vi "UHR-Fleezers Control (host) -Leonardo 04-2018 V1.vi"(0 "Tab Control":T5(tab)=enum."Trap Control (RF)") -> ()   [LabVIEW 2013] (continued)
        n483 = property on="APD Chart" class="WFChart (strict)"("YScale.Maximum"=w830) -> ()  [unwired: 2 in, 2 out]
      }
      event "Phase adj. (AI1)", "+ phase (AI1)", "- phase (AI1)": Value Change {
        n484 = event-data() -> ()  [unwired: 7 out]
        n485 = Negate(x="Phase adj. (AI1)") -> (-x=w847:i16)
        n486 = Select(t=w847, s="- phase (AI1)", f="Phase adj. (AI1)") -> (s? t:f=w846:i16)
        n487 = xnode "Read/Write Control"("FPGA VI Reference In"=w850, "error in"=w849, "Phase count adjustment"=w846) -> ("FPGA VI Reference Out"=w845:T20, "error out"=w844:errorcluster)
        n488 = Or(x="- phase (AI1)", y="+ phase (AI1)") -> (x .or. y?=w841:bool)
        n489 = xnode "Read/Write Control"("FPGA VI Reference In"=w845, "error in"=w844, "+ phase"=w841) -> ("error out"=w840:errorcluster)  [unwired: 1 out]
      }
      event "Signals to Plot": Double Click {
        w853 = u32 9868950 ("Color Box")
        n490 = event-data() -> ("Row"=w855:i32)  [unwired: 9 out]
        n491 = property on="All Signals" class="WFChart (strict)"("Active Plot"=w855) -> (error out=w866:errorcluster)  [unwired: 2 in, 1 out]
        n492 = property on="All Signals" class="WFChart (strict)" props=["Plot", "Visible?", "Plot", "Plot Color"](error in=w866) -> (error out=w865:errorcluster, "Plot.Visible?"=w864:bool)  [unwired: 1 in, 2 out]
        n493 = Select(t=FALSE ("Plot.Visible"), s=w864, f=TRUE ("Plot.Visible")) -> (s? t:f=w859:bool)
        n494 = property on="All Signals" class="WFChart (strict)"(error in=w865, "Plot.Visible?"=w859) -> (error out=w861:errorcluster)  [unwired: 1 in, 1 out]
        n495 = property on="All Signals" class="WFChart (strict)"(error in=w861) -> (error out=w856:errorcluster, "Plot.Plot Color"=w860:u32)  [unwired: 1 in, 1 out]
        n496 = property on="Signals to Plot" class="LstBox (strict)"(error in=w856, "Active Row"=w855) -> (error out=w854:errorcluster)  [unwired: 1 in, 1 out]
        n497 = Select(t=w860, s=w859, f=u32 0) -> (s? t:f=w857:u32)
        n498 = property on="Signals to Plot" class="LstBox (strict)"(error in=w854, "CellFontColor"=w857, "SelColor"=w853, "CellBG"=w853, "CellFontSize"=u32 20 ("Active Row:Cell Font:Size"), "CellFontBold"=TRUE ("Active Row:Cell Font:Bold")) -> ()  [unwired: 1 in, 2 out]
      }
      event "Dynamic Force FB": Value Change {
        n499 = event-data() -> ()  [unwired: 7 out]
        n500 = xnode "Read/Write Control"("FPGA VI Reference In"=w868, "Dynamic Force FB (Ronen)"="Dynamic Force FB") -> ()  [unwired: 1 in, 2 out]
      }
      event "BD 1 Frequency 1 (MHz)", "BD 1 Frequency 2 (MHz)", "BD 1 Frequency 3 (MHz)", "BD 2 Frequency 1 (MHz)", "BD 2 Frequency 2 (MHz)", "BD 2 Frequency 3 (MHz)", "Trap Delta (MHz)": Value Change {
        # "anytime one of the frequencies is changed, write it to the RF board UNLESS Set 2 is being oscillated. The oscillation\nscript writes the frequencies to the RF board."
        n501 = event-data() -> ("CtlRef"=w871:refnum<vi>)  [unwired: 6 out]
        n502 = control-ref of="Trap Delta (MHz)"() -> (w870:refnum<vi>)
        n503 = Equal?(x=w870, y=w871) -> (x = y?=w869:bool)
        n504 = case shown="False" "Oscillate Set 2" {
          tunnel: w874 -> [w895 _]
          tunnel: [w894 w907] -> w873
          tunnel: w872 -> [w893 w907]
          tunnel: w869 -> [w880 _]
          frame False {
            n505 = case shown="True" "Symmetric manual \ntrap motion" {
              tunnel: ["T2 for asymmetric\n(MHz)" w906] -> w881
              tunnel: "Trap Delta (MHz)" -> [w900 w905]
              tunnel: [w899 w902] -> w877
              frame False {
                n506 = Subtract(x="T2 for asymmetric\n(MHz)", y=w900) -> (x-y=w899:dbl)
              }
              frame True {
                n507 = Divide(x=w905, y=2) -> (x/y=w903:dbl)
                n508 = Subtract(x="Middle freq for \nsymmetric (MHz)", y=w903) -> (x-y=w902:dbl)
                n509 = Add(x="Middle freq for \nsymmetric (MHz)", y=w903) -> (x+y=w906:dbl)
              }
            }
            n510 = local read "BD 1 Frequency 2 (MHz)"() -> (w882:dbl)
            n511 = local write "BD 1 Frequency 1 (MHz)"(w877) -> ()
            n512 = Select(t=w881, s=w880, f=w882) -> (s? t:f=w879:dbl)
            n513 = local read "Y RF Frequency Limits (MHz)"() -> (w883:T16)
            n514 = local read "X RF Frequency Limits (MHz)"() -> (w884:T16)
            n515 = local read "BD 1 Frequency 3 (MHz)"() -> (w896:dbl)
            n516 = local write "BD 1 Frequency 2 (MHz)"(w879) -> ()
            n517 = local read "BD 2 Frequency 1 (MHz)"() -> (w887:dbl)
            n518 = local read "BD 2 Frequency 2 (MHz)"() -> (w886:dbl)
            n519 = local read "BD 2 Frequency 3 (MHz)"() -> (w897:dbl)
            n520 = call "set RF board frequency - interlace.vi"("Board 2 Frequency Limits"=w883, "Board 1 Frequency Limits"=w884, "error in"=w893, "FPGA VI Reference In"=w895, "Board 2 Frequency 3 (MHz)"=w897, "Board 1 Frequency 3 (MHz)"=w896, "Board 2 Frequency 2 (MHz)"=w886, "Board 2 Frequency 1 (MHz)"=w887, "Board 1 Frequency 2 (MHz)"=w879, "Board 1 Frequency 1  (MHz)"=w877) -> ("error out"=w894:errorcluster)  [unwired: 1 out]
            n521 = Subtract(x=w887, y=w886) -> (x-y=w891:dbl)
            n522 = Subtract(x=w879, y=w877) -> (x-y=w892:dbl)
            n523 = Square(x=w891) -> (x^2=w889:dbl)
            n524 = Square(x=w892) -> (x^2=w890:dbl)
            n525 = Add(x=w890, y=w889) -> (x+y=w888:dbl)
            n526 = Square Root(x=w888) -> (sqrt(x)=w885:dbl)
            n527 = local write "Trap Delta (MHz)"(w885) -> ()
            n528 = property on="Initial delta (MHz)" class="DigNum (strict)"("Val(Sgnl)"=w885) -> ()  [unwired: 2 in, 2 out]
          }
          frame True {
          }
        }
      }
      event "Round T1 X": Value Change {
        n529 = event-data() -> ()  [unwired: 7 out]
        n530 = local read "BD 1 Frequency 1 (MHz)"() -> (w910:dbl)
        n531 = Round To Nearest(number=w910) -> (nearest integer value=w909:dbl)
        n532 = property on="BD 1 Frequency 1 (MHz)" class="DigNum (strict)"("Val(Sgnl)"=w909) -> ()  [unwired: 2 in, 2 out]
      }
      event "Round T2 X": Value Change {
        n533 = event-data() -> ()  [unwired: 7 out]
        n534 = local read "BD 1 Frequency 2 (MHz)"() -> (w912:dbl)
        n535 = Round To Nearest(number=w912) -> (nearest integer value=w911:dbl)
        n536 = property on="BD 1 Frequency 2 (MHz)" class="DigNum (strict)"("Val(Sgnl)"=w911) -> ()  [unwired: 2 in, 2 out]
      }
      event "Stop All": Value Change {
        n537 = event-data() -> ()  [unwired: 7 out]
        n538 = call "hamilton_controller.vi"("action"=T21."DISCONNECT") -> ()  [unwired: 10 in, 1 out]
        n539 = local read "Stop All"() -> (w915:bool)
      }
      event "Delayed Interlace Start": Value Change {
        n540 = event-data() -> ()  [unwired: 7 out]
        n541 = flat-sequence {
          frame #0 {
            n542 = Multiply(x="Delay to Interlace (s)", y=1000.0) -> (x*y=w918:dbl)
            n543 = Wait (ms)(milliseconds to wait=w918) -> ()  [unwired: 1 out]
          }
          frame #1 {
            n544 = property on="Green laser mode" class="RadioBtnsControl (strict)"("Val(Sgnl)"=enum32{"Laser ON", "Laser OFF", "Interlace"}."Interlace" ("Value (Signaling)")) -> ()  [unwired: 2 in, 2 out]
          }
        }
      }
      event "BD 1 Amplitude 1 (%)", "BD 1 Amplitude 2 (%)", "BD 1 Amplitude 3 (%)", "BD 2 Amplitude 1 (%)", "BD 2 Amplitude 2 (%)", "BD 2 Amplitude 3 (%)", "Trap 1 ON", "Trap 2 ON", "Trap 3 ON", "Feedback On/Off", "All FB On/Off": Value Change {
        w942 = i16 1 ("f")
        n545 = event-data() -> ()  [unwired: 7 out]
        n546 = local write "Trap 1 (ON/OFF)"("Trap 1 ON") -> ()
        n547 = local write "Trap 2 (ON/OFF)"("Trap 2 ON") -> ()
        n548 = Boolean To (0,1)(Boolean="Trap 3 ON") -> (0, 1=w943:i16)
        n549 = Boolean To (0,1)(Boolean="Trap 1 ON") -> (0, 1=w944:i16)
        n550 = Boolean To (0,1)(Boolean="Trap 2 ON") -> (0, 1=w945:i16)
        n551 = Select(t=w945, s="Trap ON/OFF X or Y Amp?", f=w942) -> (s? t:f=w940:i16)
        n552 = Select(t=w944, s="Trap ON/OFF X or Y Amp?", f=w942) -> (s? t:f=w941:i16)
        n553 = Select(t=w943, s="Trap ON/OFF X or Y Amp?", f=w942) -> (s? t:f=w939:i16)
        n554 = Select(t=w942, s="Trap ON/OFF X or Y Amp?", f=w945) -> (s? t:f=w937:i16)
        n555 = Select(t=w942, s="Trap ON/OFF X or Y Amp?", f=w944) -> (s? t:f=w938:i16)
        n556 = Select(t=w942, s="Trap ON/OFF X or Y Amp?", f=w943) -> (s? t:f=w936:i16)
        n557 = And(x="All FB On/Off", y="Feedback On/Off") -> (x .and. y?=w934:cluster{"Set 1":bool, "Set 2":bool})
        n558 = local read "BD 1 Amplitude 1 (%)"() -> (w954:dbl)
        n559 = local read "BD 1 Amplitude 2 (%)"() -> (w953:dbl)
        n560 = local read "BD 1 Amplitude 3 (%)"() -> (w952:dbl)
        n561 = Unbundle By Name(w934) -> ("Set 1"=w930:bool, "Set 2"=w927:bool)
        n562 = local read "Y RF Amplitude Limits (%)"() -> (w923:T16)
        n563 = local read "X RF Amplitude Limits (%)"() -> (w924:T16)
        n564 = local read "BD 2 Amplitude 1 (%)"() -> (w955:dbl)
        n565 = local read "BD 2 Amplitude 2 (%)"() -> (w956:dbl)
        n566 = local read "BD 2 Amplitude 3 (%)"() -> (w957:dbl)
        n567 = And(x="Trap 2 ON", y=w927) -> (x .and. y?=w925:bool)
        n568 = And(x="Trap 1 ON", y=w930) -> (x .and. y?=w928:bool)
        n569 = Multiply(x=w941, y=w954) -> (x*y=w949:dbl)
        n570 = Multiply(x=w953, y=w940) -> (x*y=w947:dbl)
        n571 = Multiply(x=w952, y=w939) -> (x*y=w948:dbl)
        n572 = Multiply(x=w955, y=w938) -> (x*y=w958:dbl)
        n573 = Multiply(x=w956, y=w937) -> (x*y=w959:dbl)
        n574 = Multiply(x=w957, y=w936) -> (x*y=w960:dbl)
        n575 = call "set RF board amplitude - interlace.vi"("Board 2 Amplitude Limits"=w923, "Board 1 Amplitude Limits"=w924, "error in"=w950, "FPGA VI Reference In"=w951, "Board 2 Amplitude 3 (%)"=w960, "Board 1 Amplitude 3 (%)"=w948, "Board 2 Amplitude 2 (%)"=w959, "Board 2 Amplitude 1 (%)"=w958, "Board 1 Amplitude 2 (%)"=w947, "Board 1 Amplitude 1 (%)"=w949) -> ("error out"=w932:errorcluster, "FPGA VI Reference Out"=w933:T20)
        n576 = xnode "Read/Write Control"("FPGA VI Reference In"=w933, "error in"=w932, "FB On/Off Set 1"=w928, "FB On/Off Set 2"=w925) -> ("error out"=w931:errorcluster)  [unwired: 1 out]
        n577 = case shown="True" "All FB On/Off" {
          frame False {
          }
          frame True {
            n578 = local write "Feedback overload"(FALSE) -> ()
          }
        }
      }
      event "Load parameters": Value Change {
        n579 = event-data() -> ()  [unwired: 7 out]
        n580 = property on="Saved AOD Raster Scan Parameter Sets" class="Arr (strict)"() -> ("Index Values"=w972:u32[])  [unwired: 2 in, 2 out]
        n581 = Index Array(array=w972, index=0) -> (element=w969:u32)
        n582 = local write "Load parameters"(FALSE ("Load parameters")) -> ()
        n583 = Index Array(array="Saved AOD Raster Scan Parameter Sets", index=w969) -> (element=w968:T31)
        n584 = Unbundle By Name(w968) -> ("Scan Range AOD (nm) 2"=w967:dbl, "Step Size AOD (nm) 2"=w966:dbl, "Scan Speed AOD (nm/s) 2"=w965:dbl, "Number of scans (AOD) 2"=w964:u16)
        n585 = flat-sequence {
          tunnel: w967 -> [w975]
          tunnel: w966 -> [w974]
          tunnel: w965 -> [w973]
          tunnel: w964 -> [w976]
          frame #0 {
            n586 = local write "Scan Speed (nm/s)"(w973) -> ()
            n587 = local write "Scan Range (nm)"(w975) -> ()
            n588 = local write "Step Size (nm)"(w974) -> ()
          }
          frame #1 {
            n589 = property on="Number of F/B Scans (AOD)" class="DigNum (strict)"("Val(Sgnl)"=w976) -> ()  [unwired: 2 in, 2 out]
          }
        }
      }
      event "Trap 1 (ON/OFF)", "Trap 2 (ON/OFF)": Value Change {
        n590 = event-data() -> ()  [unwired: 7 out]
        n591 = property on="Trap 2 ON" class="Bool (strict)"("Val(Sgnl)"="Trap 2 (ON/OFF)") -> ()  [unwired: 2 in, 2 out]
        n592 = property on="Trap 1 ON" class="Bool (strict)"("Val(Sgnl)"="Trap 1 (ON/OFF)") -> ()  [unwired: 2 in, 2 out]
      }
      event "DIO count 1 (ticks)", "DIO count 2 (ticks)", "DIO count 3 (ticks)", "Interlace", "Number Interlace Sets", "Not-Interlacing Set": Value Change {
        n593 = event-data() -> ()  [unwired: 7 out]
        n594 = local read "DIO count 3 (ticks)"() -> (w989:u32)
        n595 = local read "DIO count 1 (ticks)"() -> (w991:u32)
        n596 = local read "DIO count 2 (ticks)"() -> (w990:u32)
        n597 = To Unsigned Byte Integer(number="Not-Interlacing Set") -> (unsigned 8bit integer=w980:u8)
        n598 = Add(x=w980, y=u8 1) -> (x+y=w984:u8)
        n599 = xnode "Read/Write Control"("FPGA VI Reference In"=w995, "error in"=w993, "DIO count 1 (ticks)"=w991, "DIO count 2 (ticks)"=w990, "DIO count 3 (ticks)"=w989, "Interlace ON/OFF"="Interlace", "Number Interlace Cycles"="Number Interlace Sets", "Interlace Off Parameters"=w984) -> ("error out"=w994:errorcluster)  [unwired: 1 out]
        n600 = Build Array(w991, w990, w989) -> (w982:u32[])
        n601 = Split 1D Array(array=w982, index="Number Interlace Sets") -> (first subarray=w992:u32[])  [unwired: 1 out]
        n602 = Index Array(array=w982, index=w980) -> (element=w981:u32)
        n603 = Add Array Elements(numeric array=w992) -> (sum=w986:u32)
        n604 = Select(t=w986, s="Interlace", f=w981) -> (s? t:f=→"Total Counts (ticks)":u32)
      }
      event "Reset Feedback": Value Change {
        n605 = event-data() -> ()  [unwired: 7 out]
        n606 = Unbundle By Name("Reset Feedback") -> ("Set 1"=w999:bool, "Set 2"=w998:bool)
        n607 = xnode "Read/Write Control"("FPGA VI Reference In"=w1001, "error in"=w996, "FB Reset Set 1"=w999, "FB Reset Set 2"=w998) -> ("error out"=w997:errorcluster)  [unwired: 1 out]
      }
      event "PID gains": Value Change {
        n608 = event-data() -> ()  [unwired: 7 out]
        n609 = local read "PID gains"() -> (w1002:T10)
        n610 = xnode "Read/Write Control"("FPGA VI Reference In"=w1005, "error in"=w1003, "FB Gains"=w1002) -> ("error out"=w1004:errorcluster)  [unwired: 1 out]
      }
      event "AI2 to Setpoint", "Trap Intensity\nSetpoints (V)": Value Change {
        n611 = event-data() -> ()  [unwired: 7 out]
        n612 = xnode "Read/Write Control"("FPGA VI Reference In"=w1010, "error in"=w1006) -> ("FPGA VI Reference Out"=w1009:T20, "error out"=w1008:errorcluster, "AI2 Y Sum Set 1"=w1017:i16, "AI2 Y Sum Set 2"=w1016:i16)
        n613 = Cluster To Array(cluster="AI2 to Setpoint") -> (array=w1020:bool[])
        n614 = local read "AI2 (V)"() -> (w1018:cluster{"Set 1":dbl, "Set 2":dbl})
        n615 = Or Array Elements(Boolean array=w1020) -> (logical OR=w1021:bool)
        n616 = Bundle By Name(cluster=w1018, "Set 1"=w1017, "Set 2"=w1016) -> (w1015:cluster{"Set 1":dbl, "Set 2":dbl})
        n617 = Divide(x=w1015, y=3276.7) -> (x/y=w1014:cluster{"Set 1":dbl, "Set 2":dbl})
        "AI2 (V)" <- w1014
        n618 = case shown="True" w1021 {
          tunnel: [w1024 w1041] -> w1013
          tunnel: "AI2 to Setpoint" -> [_ w1037]
          tunnel: "Trap Intensity\nSetpoints (V)" -> [w1025 w1040]
          tunnel: w1014 -> [_ w1034]
          frame False {
            n619 = Multiply(x=3276.7, y=w1025) -> (x*y=w1026:cluster{"Set 1":dbl, "Set 2":dbl})
            n620 = To Word Integer(number=w1026) -> (16bit integer=w1024:cluster{"Set 1":i16, "Set 2":i16})
          }
          frame True {
            n621 = Unbundle By Name(w1034) -> ("Set 1"=w1033:dbl, "Set 2"=w1032:dbl)
            n622 = Unbundle By Name(w1040) -> ("Set 1"=w1039:dbl, "Set 2"=w1038:dbl)
            n623 = Unbundle By Name(w1037) -> ("Set 1"=w1036:bool, "Set 2"=w1035:bool)
            n624 = Select(t=w1033, s=w1036, f=w1039) -> (s? t:f=w1031:dbl)
            n625 = Select(t=w1032, s=w1035, f=w1038) -> (s? t:f=w1030:dbl)
            n626 = Bundle By Name(cluster=w1040, "Set 1"=w1031, "Set 2"=w1030) -> (w1028:cluster{"Set 1":dbl, "Set 2":dbl})
            n627 = local write "Trap Intensity\nSetpoints (V)"(w1028) -> ()
            n628 = Multiply(x=3276.7, y=w1028) -> (x*y=w1029:cluster{"Set 1":dbl, "Set 2":dbl})
            n629 = To Word Integer(number=w1029) -> (16bit integer=w1041:cluster{"Set 1":i16, "Set 2":i16})
          }
        }
        n630 = Unbundle By Name(w1013) -> ("Set 1"=w1012:i16, "Set 2"=w1011:i16)
        n631 = xnode "Read/Write Control"("FPGA VI Reference In"=w1009, "error in"=w1008, "FB Setpoint Set 1"=w1012, "FB Setpoint Set 2"=w1011) -> ("error out"=w1007:errorcluster)  [unwired: 1 out]
      }
      event "Invert GI": Value Change {
        n632 = event-data() -> ()  [unwired: 7 out]
        n633 = xnode "Read/Write Control"("FPGA VI Reference In"=w1046, "error in"=w1044, "Invert GI"="Invert GI", "Invert GI 2"="Invert GI") -> ("error out"=w1045:errorcluster)  [unwired: 1 out]
      }
      event "Green FB Setpoint (mV)", "Green FB Gains", "Green FB On/Off", "Current When FB OFF (%)", "Green int current ON count adj": Value Change {
        n634 = event-data() -> ()  [unwired: 7 out]
        n635 = local read "Green FB Setpoint (mV)"() -> (w1053:dbl)
        n636 = local read "Current When FB OFF (%)"() -> (w1056:dbl)
        n637 = Multiply(x=w1053, y=3.2767) -> (x*y=w1052:dbl)
        n638 = Multiply(x=w1056, y=655.35) -> (x*y=w1057:dbl)
        n639 = To Unsigned Word Integer(number=w1057) -> (unsigned 16bit integer=w1055:u16)
        n640 = local read "Green int current ON count adj"() -> (w1060:u32)
        n641 = local read "Green FB Gains"() -> (w1059:T10)
        n642 = local read "Green Laser ON/Interlacing"() -> (w1050:bool)
        n643 = local read "Green laser mode"() -> (w1049:enum32{"Laser ON", "Laser OFF", "Interlace"})
        n644 = local read "Green FB On/Off"() -> (w1061:bool)
        n645 = Equal?(x=w1049, y=enum32{"Laser ON", "Laser OFF", "Interlace"}."Interlace") -> (x = y?=w1047:bool)
        n646 = Compound Arithmetic op=AND(w1047, w1061, w1050) -> (w1051:bool)
        n647 = xnode "Read/Write Control"("FPGA VI Reference In"=w1064, "error in"=w1063, "Green FB Setpoint"=w1052, "Green FB On/Off"=w1051, "Current Out"=w1055, "Green int current ON count adj"=w1060, "Green FB Gains"=w1059) -> ("error out"=w1062:errorcluster)  [unwired: 1 out]
      }
      event "Green laser mode", "Green Laser ON/Interlacing": Value Change {
        n648 = event-data() -> ()  [unwired: 7 out]
        n649 = case shown="True" "Green Laser ON/Interlacing" {
          tunnel: "Green laser mode" -> [_ w1078]
          tunnel: [enum32{"Laser ON", "Laser OFF", "Interlace"}."Laser OFF" ("Green laser mode") w1078] -> w1066
          tunnel: [FALSE w1074] -> w1065
          frame False {
          }
          frame True {
            n650 = local read "Green FB On/Off"() -> (w1075:bool)
            n651 = Equal?(x=w1078, y=enum32{"Laser ON", "Laser OFF", "Interlace"}."Interlace") -> (x = y?=w1076:bool)
            n652 = And(x=w1076, y=w1075) -> (x .and. y?=w1074:bool)
          }
        }
        n653 = xnode "Read/Write Control"("FPGA VI Reference In"=w1071, "error in"=w1069, "Operating Mode"=w1066, "Operating Mode 2"=w1066, "Green FB On/Off"=w1065) -> ("error out"=w1070:errorcluster)  [unwired: 1 out]
      }
      event "- phase (APD 1 Gate)", "+ phase (APD 1 Gate)": Value Change {
        n654 = event-data() -> ()  [unwired: 7 out]
        n655 = local read "Phase Adj. (APD 1 Gate)"() -> (w1079:i16)
        n656 = Negate(x=w1079) -> (-x=w1087:i16)
        n657 = Select(t=w1087, s="- phase (APD 1 Gate)", f=w1079) -> (s? t:f=w1086:i16)
        n658 = Or(x="- phase (APD 1 Gate)", y="+ phase (APD 1 Gate)") -> (x .or. y?=w1082:bool)
        n659 = xnode "Read/Write Control"("FPGA VI Reference In"=w1089, "error in"=w1088, "Phase count adjustment (APD 1 Gate)"=w1086) -> ("FPGA VI Reference Out"=w1084:T20, "error out"=w1085:errorcluster)
        n660 = xnode "Read/Write Control"("FPGA VI Reference In"=w1084, "error in"=w1085, "+ phase (APD 1 Gate)"=w1082) -> ("error out"=w1083:errorcluster)  [unwired: 1 out]
      }
      event "+ phase (APD 2 Gate)", "- phase (APD 2 Gate)": Value Change {
        n661 = event-data() -> ()  [unwired: 7 out]
        n662 = local read "Phase Adj. (APD 2 Gate)"() -> (w1090:i16)
        n663 = Negate(x=w1090) -> (-x=w1098:i16)
        n664 = Select(t=w1098, s="- phase (APD 2 Gate)", f=w1090) -> (s? t:f=w1097:i16)
        n665 = Or(x="- phase (APD 2 Gate)", y="+ phase (APD 2 Gate)") -> (x .or. y?=w1093:bool)
        n666 = xnode "Read/Write Control"("FPGA VI Reference In"=w1100, "error in"=w1099, "Phase count adjustment (APD 2 Gate)"=w1097) -> ("FPGA VI Reference Out"=w1095:T20, "error out"=w1096:errorcluster)
        n667 = xnode "Read/Write Control"("FPGA VI Reference In"=w1095, "error in"=w1096, "+ phase (APD 2 Gate)"=w1093) -> ("error out"=w1094:errorcluster)  [unwired: 1 out]
      }
      event "Phase Adj. (APD Acq)", "+ phase (APD Acq)", "- phase (APD Acq)": Value Change {
        n668 = event-data() -> ()  [unwired: 7 out]
        n669 = local read "Phase Adj. (APD Acq)"() -> (w1103:i16)
        n670 = Negate(x=w1103) -> (-x=w1109:i16)
        n671 = Select(t=w1109, s="+ phase (APD Acq)", f=w1103) -> (s? t:f=w1108:i16)
        n672 = Or(x="+ phase (APD Acq)", y="- phase (APD Acq)") -> (x .or. y?=w1104:bool)
        n673 = xnode "Read/Write Control"("FPGA VI Reference In"=w1111, "error in"=w1110, "Phase Count Adjustment (APD Acq)"=w1108) -> ("FPGA VI Reference Out"=w1106:T20, "error out"=w1107:errorcluster)
        n674 = xnode "Read/Write Control"("FPGA VI Reference In"=w1106, "error in"=w1107, "+ phase (APD Acq)"=w1104) -> ("error out"=w1105:errorcluster)  [unwired: 1 out]
      }
      event "Phase adj. (GI)", "+ phase (GI)", "- phase (GI)": Value Change {
        n675 = event-data() -> ()  [unwired: 7 out]
        n676 = Negate(x="Phase adj. (GI)") -> (-x=w1120:i16)
        n677 = Select(t=w1120, s="+ phase (GI)", f="Phase adj. (GI)") -> (s? t:f=w1119:i16)
        n678 = Or(x="+ phase (GI)", y="- phase (GI)") -> (x .or. y?=w1115:bool)
        n679 = xnode "Read/Write Control"("FPGA VI Reference In"=w1122, "error in"=w1121, "Phase count adjustment (GI)"=w1119) -> ("FPGA VI Reference Out"=w1117:T20, "error out"=w1118:errorcluster)
        n680 = xnode "Read/Write Control"("FPGA VI Reference In"=w1117, "error in"=w1118, "+ phase (GI)"=w1115) -> ("error out"=w1116:errorcluster)  [unwired: 1 out]
      }
      event "Phase adj. (GI) 2", "+ phase (GI) 2", "- phase (GI) 2": Value Change {
        n681 = event-data() -> ()  [unwired: 7 out]
        n682 = Negate(x="Phase adj. (GI) 2") -> (-x=w1131:i16)
        n683 = Select(t=w1131, s="+ phase (GI) 2", f="Phase adj. (GI) 2") -> (s? t:f=w1130:i16)
        n684 = Or(x="+ phase (GI) 2", y="- phase (GI) 2") -> (x .or. y?=w1126:bool)
        n685 = xnode "Read/Write Control"("FPGA VI Reference In"=w1133, "error in"=w1132, "Phase count adjustment (GI) 2"=w1130) -> ("FPGA VI Reference Out"=w1128:T20, "error out"=w1129:errorcluster)
        n686 = xnode "Read/Write Control"("FPGA VI Reference In"=w1128, "error in"=w1129, "+ phase (GI) 2"=w1126) -> ("error out"=w1127:errorcluster)  [unwired: 1 out]
      }
      event "Phase adj. (Green FB)", "- phase (Green FB)", "+ phase (Green FB)": Value Change {
        n687 = event-data() -> ()  [unwired: 7 out]
        n688 = Negate(x="Phase adj. (Green FB)") -> (-x=w1142:i16)
        n689 = Select(t=w1142, s="+ phase (Green FB)", f="Phase adj. (Green FB)") -> (s? t:f=w1141:i16)
        n690 = Or(x="+ phase (Green FB)", y="- phase (Green FB)") -> (x .or. y?=w1137:bool)
        n691 = xnode "Read/Write Control"("FPGA VI Reference In"=w1144, "error in"=w1143, "Phase count adjustment (Green FB)"=w1141) -> ("FPGA VI Reference Out"=w1139:T20, "error out"=w1140:errorcluster)
        n692 = xnode "Read/Write Control"("FPGA VI Reference In"=w1139, "error in"=w1140, "+ phase (Green FB)"=w1137) -> ("error out"=w1138:errorcluster)  [unwired: 1 out]
      }
      event "Invert APD Gate", "APD Gate ON Count", "APD Gate OFF Count", "APD Gate", "APD Integration Time (s)", "APD 1 AO Mult.", "APD 2 AO Mult.": Value Change {
        n693 = event-data() -> ()  [unwired: 7 out]
        n694 = local read "APD Integration Time (s)"() -> (w1145:dbl)
        n695 = local read "APD Gate ON Count"() -> (w1158:u32)
        n696 = local read "APD Gate OFF Count"() -> (w1157:u32)
        n697 = local read "Invert APD Gate"() -> (w1159:bool)
        n698 = local read "APD Gate"() -> (w1156:enum32{"ON", "OFF", "Interlace"})
        n699 = Multiply(x=w1145, y=40000000.0) -> (x*y=w1154:dbl)
        n700 = Reciprocal(x=w1145) -> (1/x=→"APD Acq Rate (Hz)":dbl)
        n701 = To Unsigned Long Integer(number=w1154) -> (unsigned 32bit integer=w1153:u32)
        n702 = local read "DMA Update Period (s)"() -> (w1146:dbl)
        n703 = Divide(x=w1146, y=w1145) -> (x/y=w1149:dbl)
        n704 = local read "APD 1 AO Mult."() -> (w1151:i16)
        n705 = local read "APD 2 AO Mult."() -> (w1150:i16)
        n706 = Multiply(x=2.0, y=w1149) -> (x*y=w1148:dbl)
        n707 = local write "APD Samples/FIFO Acq."(w1149) -> ()
        n708 = local write "APD Elements/DMA read"(w1148) -> ()
        n709 = xnode "Read/Write Control"("FPGA VI Reference In"=w1162, "error in"=w1161, "Invert APD Gate"=w1159, "APD Gate ON Count"=w1158, "APD Gate OFF Count"=w1157, "APD Acq Rate Count"=w1153, "APD Gate Operating Mode"=w1156, "APD 1 AO scale factor"=w1151, "APD 2 AO scale factor"=w1150) -> ("error out"=w1160:errorcluster)  [unwired: 1 out]
      }
      event "GI Frequency, ON count", "Green FB Count", "GI Frequency, OFF count": Value Change {
        n710 = event-data() -> ()  [unwired: 7 out]
        n711 = xnode "Read/Write Control"("FPGA VI Reference In"=w1168, "error in"=w1166, "Green interlace ON count"="GI Frequency, ON count", "Green interlace OFF count"="GI Frequency, OFF count", "Green interlace ON count 2"="GI Frequency, ON count", "Green interlace OFF count 2"="GI Frequency, OFF count", "Green FB Count"="Green FB Count") -> ("error out"=w1167:errorcluster)  [unwired: 1 out]
      }
      event "Number of F/B Scans (AOD)", "Scan Speed (nm/s)", "Scan BD", "Initial delta (MHz)", "Step Size (nm)", "Scan Range (nm)": Value Change {
        w1230 = 123.0  # AOM cal (nm/MHz)
        n712 = event-data() -> ()  [unwired: 7 out]
        n713 = local read "BD 1 Frequency 1 (MHz)"() -> (w1213:dbl)
        n714 = local read "AOM X Cal (nm/MHz)"() -> (w1205:dbl)
        n715 = local read "X RF Frequency Limits (MHz)"() -> (w1217:T16)
        n716 = local read "Y RF Frequency Limits (MHz)"() -> (w1214:T16)
        n717 = local read "BD 2 Frequency 1 (MHz)"() -> (w1219:dbl)
        n718 = Negate(x="Scan Range (nm)") -> (-x=w1183:dbl)
        n719 = Divide(x=w1183, y=w1205) -> (x/y=w1187:dbl)
        n720 = Select(t=w1217, s="Scan BD", f=w1214) -> (s? t:f=w1216:T16)
        n721 = Select(t=w1213, s="Scan BD", f=w1219) -> (s? t:f=w1218:dbl)
        n722 = Unbundle By Name(w1216) -> ("Maximum"=w1225:dbl, "Minimum"=w1224:dbl)
        n723 = Add(x=w1187, y=w1218) -> (x+y=w1222:dbl)
        n724 = Divide(x=w1183, y="Step Size (nm)") -> (x/y=w1202:dbl)
        n725 = Divide(x="Step Size (nm)", y=w1205) -> (x/y=w1211:dbl)
        n726 = Absolute Value(x=w1202) -> (abs(x)=w1186:dbl)
        n727 = Sign(1:w1183) -> (0:w1184:dbl)
        n728 = In Range and Coerce(upper limit=w1225, x=w1222, lower limit=w1224) -> (coerced(x)=w1221:dbl, In Range?=w1223:bool)
        n729 = To Unsigned Quad Integer(1:w1186) -> (0:w1201:u64)
        "Scan steps (AOD)" <- w1201
        n730 = call "IR AOM freq to word.vi"("Frequency In (MHz)"=w1211) -> ("Frequency Word Out (double)"=w1208:dbl)
        n731 = Multiply(x=w1184, y=w1208) -> (x*y=w1185:dbl)
        n732 = Subtract(x=w1222, y=w1221) -> (x-y=w1220:dbl)
        n733 = To Quad Integer(1:w1185) -> (0:w1207:i64)
        "Incr. int (AOD)" <- w1207
        n734 = Subtract(x=w1187, y=w1220) -> (x-y=w1206:dbl)
        "Scan Range (MHz)" <- w1206
        n735 = Select(t=w1187, s=w1223, f=w1206) -> (s? t:f=w1226:dbl)
        n736 = Multiply(x=w1206, y=w1205) -> (x*y=w1204:dbl)
        n737 = Decrement(x=w1201) -> (x-1=w1254:u64)
        n738 = Negate(x=w1204) -> (-x=w1200:dbl)
        n739 = local write "Scan Range (nm)"(w1200) -> ()
        n740 = Divide(x=w1226, y=w1254) -> (x/y=w1210:dbl)
        "Scan Increment (MHz)" <- w1210
        n741 = call "IR AOM freq to word.vi"("Frequency In (MHz)"=w1210) -> ("Frequency Word Out (double)"=w1209:dbl)
        n742 = Divide(x="Step Size (nm)", y="Scan Speed (nm/s)") -> (x/y=w1197:dbl)
        n743 = To Quad Integer(1:w1209) -> ()  [unwired: 1 out]
        n744 = local read "Number Interlace Sets"() -> (w1181:u8)
        n745 = local read "AI Count (ticks)"() -> (w1182:u32)
        n746 = local read "Total Counts (ticks)"() -> (w1180:u32)
        n747 = local read "# Samples/trap"() -> (w1212:u32)
        n748 = Multiply(x=w1182, y=w1181) -> (x*y=w1179:u32)
        n749 = Divide(x=w1180, y=w1179) -> (x/y=w1178:dbl)
        n750 = Select(t=w1213, s="Scan BD", f=w1219) -> (s? t:f=w1251:dbl)
        "Initial freq. (MHz)" <- w1251
        n751 = Add(x=w1226, y=w1251) -> (x+y=→"Final freq. (MHz)":dbl)
        n752 = Divide(x=w1180, y=40000000.0) -> (x/y=w1196:dbl)
        n753 = Divide(x=w1197, y=w1196) -> (x/y=w1195:dbl)
        n754 = To Unsigned Quad Integer(1:w1195) -> (0:w1170:u64)
        n755 = Quotient & Remainder(x=w1170, y=u64 2) -> (x-y*floor(x/y)=w1174:u64)  [unwired: 1 out]
        n756 = Equal?(x=w1174, y=u64 0) -> (x = y?=w1172:bool)
        n757 = Decrement(x=w1170) -> (x-1=w1171:u64)
        n758 = Select(t=w1170, s=w1172, f=w1171) -> (s? t:f=w1169:u64)
        "Cycles/step (AOD)" <- w1169
        n759 = xnode "Read/Write Control"("FPGA VI Reference In"=w1262, "error in"=w1261, "Scan steps"=w1201, "Number of scans"="Number of F/B Scans (AOD)", "Cycles per step"=w1169, "Scan freq.  increment"=w1207, "Scan BD"="Scan BD") -> ("error out"=w1260:errorcluster)  [unwired: 1 out]
        n760 = Multiply(x=w1201, y=w1169) -> (x*y=w1255:u64)
        n761 = Multiply(x=w1255, y=u64 2) -> (x*y=w1177:u64)
        n762 = Multiply(x=w1178, y=w1177) -> (x*y=w1176:dbl)
        "Data points/scan (f/b)" <- w1176
        n763 = Multiply(x=w1176, y="Number of F/B Scans (AOD)") -> (x*y=w1258:dbl)
        "Data points/scans" <- w1258
        n764 = Divide(x=w1258, y=w1212) -> (x/y=→"N sets should be saved":dbl)
        n765 = Multiply(x=w1255, y=w1196) -> (x*y=w1194:dbl)
        "Time/Scan (s) (AOD)" <- w1194
        n766 = Select(t=w1226, s="Scan BD", f=0.0) -> (s? t:f=w1252:dbl)
        n767 = Select(t=0.0, s="Scan BD", f=w1226) -> (s? t:f=w1248:dbl)
        n768 = local read "BD 2 Frequency 2 (MHz)"() -> (w1244:dbl)
        n769 = local read "BD 1 Frequency 2 (MHz)"() -> (w1247:dbl)
        n770 = Add(x=w1248, y=w1219) -> (x+y=w1245:dbl)
        n771 = Add(x=w1213, y=w1252) -> (x+y=w1246:dbl)
        n772 = Multiply(x=w1194, y=2.0) -> (x*y=w1193:dbl)
        n773 = Multiply(x=w1193, y="Number of F/B Scans (AOD)") -> (x*y=w1190:dbl)
        n774 = Divide(x=w1190, y=60.0) -> (x/y=→"Time to Finish All (min)":dbl)
        n775 = Add(x="Trap 2 Bead Size (nm)", y="Trap 1 Bead Size (nm)") -> (x+y=w1234:dbl)
        n776 = local read "Initial delta (MHz)"() -> (w1231:dbl)
        n777 = Divide(x=w1234, y=2.0) -> (x/y=w1228:dbl)
        n778 = Subtract(x=w1245, y=w1244) -> (x-y=w1242:dbl)
        n779 = Subtract(x=w1246, y=w1247) -> (x-y=w1243:dbl)
        n780 = Square(x=w1242) -> (x^2=w1241:dbl)
        n781 = Square(x=w1243) -> (x^2=w1240:dbl)
        n782 = Add(x=w1240, y=w1241) -> (x+y=w1239:dbl)
        n783 = Square Root(x=w1239) -> (sqrt(x)=w1238:dbl)
        "Final delta (MHz)" <- w1238
        n784 = Multiply(x=w1230, y=w1238) -> (x*y=w1237:dbl)
        n785 = Multiply(x=w1231, y=w1230) -> (x*y=w1229:dbl)
        n786 = Subtract(x=w1229, y=w1228) -> (x-y=→"Initial sep (nm)":dbl)
        n787 = Subtract(x=w1237, y=w1228) -> (x-y=→"Final sep (nm)":dbl)
      }
      event "Raster Scanning...": Value Change {
        n788 = event-data() -> ("NewVal"=w1263:bool)  [unwired: 6 out]
        n789 = case shown="True" w1263 {
          frame False {
          }
          frame True {
            n790 = property on="BD 1 Frequency 1 (MHz)" class="DigNum (strict)"("Val(Sgnl)"=65.0 ("Value (Signaling)")) -> ()  [unwired: 2 in, 2 out]
          }
        }
      }
      event "Phase increment trap 1", "Swap F1 and F2", "Freq switch delay", "Amp switch delay", "Phase increment trap 2", "RF phase reset before cycles", "Phase offset method": Value Change {
        n791 = event-data() -> ()  [unwired: 7 out]
        n792 = local read "Amp switch delay"() -> (w1269:u16)
        n793 = local read "Phase increment trap 1"() -> (w1268:fxp<+/-,64,32>)
        n794 = local read "Freq switch delay"() -> (w1271:u16)
        n795 = local read "Phase increment trap 2"() -> (w1267:fxp<+/-,64,32>)
        n796 = local read "RF phase reset before cycles"() -> (w1266:bool)
        n797 = local read "Swap F1 and F2"() -> (w1270:bool)
        n798 = local read "Phase offset method"() -> (w1265:u8)
        n799 = xnode "Read/Write Control"("FPGA VI Reference In"=w1274, "error in"=w1273, "BD 1 Delay (ticks)"=w1271, "Swap F1 and F2"=w1270, "Amp switch delay"=w1269, "Phase Trap 1"=w1268, "Phase Trap 2"=w1267, "RF phase reset before cycles"=w1266, "Phase offset method"=w1265) -> ("error out"=w1272:errorcluster)  [unwired: 1 out]
      }
      event "Scan steps (MCL)", "Number of scans (MCL)", "Scan Range (V)\n(of steps)", "2D or 1D Scan", "N APD Samp/step", "Fast Scan Dir", "Continuous MCL Scanning", "Scan lines (y)": Value Change {
        w1276 = 32767.0 ("y")
        n800 = event-data() -> ()  [unwired: 7 out]
        n801 = Select(t="Scan lines (y)", s="2D or 1D Scan", f="Number of scans (MCL)") -> (s? t:f=w1281:u64)
        n802 = Decrement(x="Scan steps (MCL)") -> (x-1=w1297:u64)
        n803 = Divide(x="Scan Range (V)\n(of steps)", y=w1297) -> (x/y=w1296:dbl)
        "Desired Scan Incr (V)" <- w1296
        n804 = local read "APD Integration Time (s)"() -> (w1289:dbl)
        n805 = Multiply(x=w1296, y=w1276) -> (x*y=w1305:dbl)
        n806 = Divide(x=w1305, y=10.0) -> (x/y=w1295:dbl)
        "Desired incr (int)" <- w1295
        n807 = local read "Update Count (MCL)"() -> (w1301:u32)
        n808 = Round Toward -Infinity(1:w1295) -> (0:w1304:dbl)
        n809 = To Word Integer(number=w1304) -> (16bit integer=w1279:i16)
        "Actual Incr. int (MCL)" <- w1279
        n810 = Multiply(x=w1289, y=40000000.0) -> (x*y=w1302:dbl)
        n811 = Divide(x=w1302, y=w1301) -> (x/y=w1300:dbl)
        n812 = Multiply(x=i16 10, y=w1279) -> (x*y=w1277:i16)
        n813 = Multiply(x="N APD Samp/step", y=w1300) -> (x*y=w1299:dbl)
        "Cycles/step (MCL)" <- w1299
        n814 = Divide(x=w1277, y=w1276) -> (x/y=→"Actual MCL Inc (V)":dbl)
        n815 = Multiply(x="N APD Samp/step", y="Scan steps (MCL)") -> (x*y=w1291:dbl)
        n816 = local read "APD Samples/FIFO Acq."() -> (w1288:dbl)
        n817 = Multiply(x=w1291, y=u64 2) -> (x*y=w1290:dbl)
        "Data points/scan (f+b)" <- w1290
        n818 = Multiply(x=w1290, y=w1281) -> (x*y=w1308:dbl)
        "Data points/scans (MCL)" <- w1308
        n819 = Multiply(x=w1289, y=w1290) -> (x*y=w1282:dbl)
        "Time/f+b scan (s) (MCL)" <- w1282
        n820 = Divide(x=w1308, y=w1288) -> (x/y=→"N sets should be saved (MCL)":dbl)
        n821 = Multiply(x=w1282, y=w1281) -> (x*y=→"Total Time (s)":dbl)
        n822 = Not(x="Fast Scan Dir") -> (.not. x?=w1286:bool)
        n823 = xnode "Read/Write Control"("FPGA VI Reference In"=w1312, "error in"=w1311, "Scan steps (MCL)"="Scan steps (MCL)", "Number of scans (MCL)"=w1281, "Cycles per step (MCL)"=w1299, "Scan freq.  increment (MCL)"=w1279, "1D or 2D Scan?"="2D or 1D Scan", "MCL Scan Axis"=w1286, "Cont. Scan (MCL)"="Continuous MCL Scanning") -> ("error out"=w1310:errorcluster)  [unwired: 1 out]
      }
      event "Read Cal": Value Change {
        w1349 = 1000.0 ("y")
        w1337 = T30."big-endian, network order" ("byte order (0:big-endian, network order)")
        w1338 = -1 ("count (1)")
        n824 = event-data() -> ()  [unwired: 7 out]
        n825 = local read "Save file name"() -> (w1367:path)
        n826 = local write "Read Cal"(FALSE ("Read Cal")) -> ()
        n827 = Strip Path(path=w1367) -> (stripped path=w1366:path)  [unwired: 1 out]
        n828 = Path To String(path=w1366) -> (string=w1347:string)
        n829 = Concatenate Strings(w1347, "\\current.off" ("string")) -> (w1345:string)
        n830 = Concatenate Strings(w1347, "\\current.cal" ("string")) -> (w1364:string)
        n831 = local read "Scale intensities"() -> (w1317:bool)
        n832 = String To Path(string=w1364) -> (path=w1363:path)
        n833 = String To Path(string=w1345) -> (path=w1344:path)
        n834 = Open/Create/Replace File(file path (use dialog)=w1363, operation (0:open)=T24."open", access (0:read/write)=enum16{"read/write", "read-only", "write-only"}."read-only") -> (refnum out=w1370:refnum<file>, error out=w1359:errorcluster)  [unwired: 1 in, 3 out]
        n835 = Deny Access(4:w1359, 7:w1370) -> (0:w1358:errorcluster, 3:w1362:refnum<file>)  [unwired: 1 out]
        n836 = Open/Create/Replace File(file path (use dialog)=w1344, operation (0:open)=T24."open", access (0:read/write)=enum16{"read/write", "read-only", "write-only"}."read-only") -> (refnum out=w1341:refnum<file>)  [unwired: 1 in, 4 out]
        n837 = Deny Access(7:w1341) -> (3:w1339:refnum<file>)  [unwired: 1 in, 2 out]
        n838 = Read from Binary File(5:0.0, 8:w1358, 9:w1337, 10:w1338, 11:w1362) -> (0:w1357:errorcluster, 2:w1355:dbl[], 3:w1360:refnum<file>)  [unwired: 2 out]
        n839 = Array To Cluster(array=w1355) -> (cluster=w1354:T32)
        n840 = Unbundle(w1354) -> ("[0]"=w1328:dbl, "[1]"=w1327:dbl, "[2]"=w1314:dbl, "[3]"=w1316:dbl, "[4]"=w1353:dbl, "[5]"=w1352:dbl)
        n841 = case "Cal is OK if you load a cal with scale intensities on - Alex 081418" shown="False" w1317 {
          tunnel: w1316 -> [w1372 w1375]
          tunnel: [w1372 w1374] -> w1315
          tunnel: w1314 -> [w1371 w1377]
          tunnel: [w1371 w1376] -> w1313
          frame False {
          }
          frame True {
            n842 = local read "Scale factor"() -> (w1373:dbl)
            n843 = Multiply(x=w1375, y=w1373) -> (x*y=w1374:dbl)
            n844 = Multiply(x=w1377, y=w1373) -> (x*y=w1376:dbl)
          }
        }
        n845 = Close File(refnum=w1360, error in=w1357) -> (error out=→"Read cal error":errorcluster)  [unwired: 1 out]
        n846 = Multiply(x=w1352, y=w1349) -> (x*y=w1350:dbl)
        n847 = local write "T2 kappa_x (pN/nm)"(w1315) -> ()
        n848 = local write "T1 kappa_x (pN/nm)"(w1313) -> ()
        n849 = local write "T1 alpha_x (nm/V)"(w1328) -> ()
        n850 = local write "T2 alpha_x (nm/V)"(w1327) -> ()
        n851 = Read from Binary File(5:0.0, 9:w1337, 10:w1338, 11:w1339) -> (2:w1333:dbl[], 3:w1336:refnum<file>)  [unwired: 1 in, 3 out]
        n852 = Multiply(x=w1353, y=w1349) -> (x*y=w1351:dbl)
        n853 = local write "T1 offset_x (mV)"(w1351) -> ()
        n854 = local write "T2 offset_x (mV)"(w1350) -> ()
        n855 = Close File(refnum=w1336) -> ()  [unwired: 1 in, 2 out]
        n856 = Array Subset(array=w1333, index=3) -> (w1331:dbl[])  [unwired: 1 in]
        n857 = Index Array(array=w1333, index=0) -> (element=→"Offset file step size":dbl)
        n858 = Multiply(x=w1328, y=w1314) -> (x*y=w1325:dbl)
        n859 = Multiply(x=w1327, y=w1316) -> (x*y=w1326:dbl)
        n860 = Divide(x=w1326, y=w1325) -> (x/y=w1319:dbl)
        n861 = Decimate 1D Array(w1331) -> (w1323:dbl[], w1324:dbl[])  [unwired: 1 out]
        n862 = disable-structure "Removed B factor to improve position FB -Alex 081418 2of3" shown="Enabled" {
          disable-tunnel: w1319 -> [w1378 _]
          disable-tunnel: [w1378 1.0] -> w1318
          frame Disabled {
          }
          frame Enabled {
          }
        }
        n863 = Bundle By Name(cluster="Offset Values", "Trap 1X offset"=w1323, "Trap 2X offset"=w1324) -> (w1329:T14)
        n864 = Multiply(x=w1324, y=w1318) -> (x*y=w1322:dbl[])
        n865 = Subtract(x=w1323, y=w1322) -> (x-y=w1321:dbl[])
        n866 = local write "Offset Values"(w1329) -> ()
        n867 = case shown="True" "Auto read offset\ncorrection" {
          tunnel: w1321 -> [_ w1380]
          frame False {
          }
          frame True {
            n868 = property on="Setpoint offset\nCorrection values" class="Arr (strict)"("Val(Sgnl)"=w1380) -> ()  [unwired: 2 in, 2 out]
          }
        }
        n869 = property on="B factor" class="DigNum (strict)"("Val(Sgnl)"=w1318) -> ()  [unwired: 2 in, 2 out]
      }
      event "Abort MCL Scan": Value Change {
        n870 = event-data() -> ()  [unwired: 7 out]
        n871 = local write "MCL Scanning"(FALSE ("MCL Scanning")) -> ()
        n872 = xnode "Read/Write Control"("FPGA VI Reference In"=w1385, "error in"=w1384, "Abort scan (MCL)"="Abort MCL Scan") -> ("error out"=w1383:errorcluster)  [unwired: 1 out]
      }
      event "Update Count (MCL)": Value Change {
        n873 = event-data() -> ()  [unwired: 7 out]
        n874 = xnode "Read/Write Control"("FPGA VI Reference In"=w1389, "error in"=w1388, "MCL count"="Update Count (MCL)") -> ("error out"=w1387:errorcluster)  [unwired: 1 out]
      }
      event "Phase adjust (MCL)", "+ phase (MCL)", "- phase (MCL)": Value Change {
        n875 = event-data() -> ()  [unwired: 7 out]
        n876 = Negate(x="Phase adjust (MCL)") -> (-x=w1398:i16)
        n877 = Select(t=w1398, s="- phase (MCL)", f="Phase adjust (MCL)") -> (s? t:f=w1396:i16)
        n878 = Or(x="- phase (MCL)", y="+ phase (MCL)") -> (x .or. y?=w1391:bool)
        n879 = xnode "Read/Write Control"("FPGA VI Reference In"=w1400, "error in"=w1399, "Phase count adjustment (MCL)"=w1396) -> ("FPGA VI Reference Out"=w1392:T20, "error out"=w1393:errorcluster)
        n880 = xnode "Read/Write Control"("FPGA VI Reference In"=w1392, "error in"=w1393, "+ phase (MCL)"=w1391) -> ("error out"=w1390:errorcluster)  [unwired: 1 out]
      }
      event "Abort AOD Scan": Value Change {
        n881 = event-data() -> ()  [unwired: 7 out]
        n882 = flat-sequence {
          tunnel: w1405 -> [w1412]
          tunnel: w1404 -> [w1411]
          tunnel: [w1410] -> w1402
          tunnel: [w1406] -> w1401
          tunnel: [w1425] -> w1403
          tunnel: w1402 -> [w1425]
          tunnel: w1401 -> [w1424]
          frame #0 {
            n883 = local read "Save scans"() -> (w1408:bool)
            n884 = xnode "Read/Write Control"("FPGA VI Reference In"=w1412, "error in"=w1411, "Abort scan"="Abort AOD Scan") -> ("FPGA VI Reference Out"=w1406:T20, "error out"=w1410:errorcluster)
            n885 = local write "Raster Scanning..."(FALSE) -> ()
            n886 = case shown="True" w1408 {
              frame False {
              }
              frame True {
                n887 = local write "Stop Saving"(TRUE) -> ()
              }
            }
          }
          frame #1 {
            n888 = xnode "Read/Write Control"("FPGA VI Reference In"=w1424) -> ("BD1 Frequency Out 1"=w1415:u64)  [unwired: 1 in, 2 out]
            n889 = To Double Precision Float(number=w1415) -> (double precision float=w1421:dbl)
            n890 = Multiply(x=49125000.0, y=6.0) -> (x*y=w1420:dbl)
            n891 = Multiply(x=w1421, y=w1420) -> (x*y=w1418:dbl)
            n892 = Scale By Power Of 2(n=-48, x=w1418) -> (x*2^n=w1417:dbl)
            n893 = Divide(x=w1417, y=1000000.0) -> (x/y=w1414:dbl)
            n894 = property on="BD 1 Frequency 1 (MHz)" class="DigNum (strict)"("Val(Sgnl)"=w1414) -> ()  [unwired: 2 in, 2 out]
          }
        }
      }
      event "Continuous AOD Scanning": Value Change {
        n895 = event-data() -> ()  [unwired: 7 out]
        n896 = xnode "Read/Write Control"("FPGA VI Reference In"=w1429, "error in"=w1428, "Cont. Scan"="Continuous AOD Scanning") -> ("error out"=w1427:errorcluster)  [unwired: 1 out]
      }
      event "Index": Value Change {
        n897 = event-data() -> ()  [unwired: 7 out]
        n898 = call "Create new save file.vi"("Insert"="", "Ext"=".dat" ("string"), "Index In"="Index") -> ("Path Out"=→"Save file name":path, "Index Out"=w1430:dbl)
        "Save index" <- w1430
        n899 = local write "Index"(w1430) -> ()
      }
      event "AO1", "AO2": Value Change {
        w1445 = 10.0 ("y")
        w1444 = 32767.0 ("y")
        n900 = event-data() -> ()  [unwired: 7 out]
        n901 = local read "AO2"() -> (w1443:dbl)
        n902 = local read "AO1"() -> (w1440:dbl)
        n903 = Multiply(x=w1440, y=w1444) -> (x*y=w1439:dbl)
        n904 = Multiply(x=w1443, y=w1444) -> (x*y=w1442:dbl)
        n905 = Divide(x=w1439, y=w1445) -> (x/y=w1438:dbl)
        n906 = Divide(x=w1442, y=w1445) -> (x/y=w1441:dbl)
        n907 = To Word Integer(number=w1438) -> (16bit integer=w1446:i16)
        n908 = To Word Integer(number=w1441) -> (16bit integer=w1447:i16)
        n909 = xnode "Read/Write Control"("FPGA VI Reference In"=w1437, "error in"=w1436, "AO1 (Y)"=w1446, "AO2 (X)"=w1447) -> ("error out"=w1435:errorcluster)  [unwired: 1 out]
      }
      event "Inject Top:": Value Change {
        n910 = event-data() -> ()  [unwired: 7 out]
        n911 = disable-structure shown="Enabled" {
          disable-tunnel: "Inject Top:" -> [w1449 w1489]
          frame Disabled {
            n912 = local read "Chemyx Syringe Pump Serial Port"() -> (w1450:refnum<visa-resource-name>)
            n913 = local read "Pump write delay (ms)"() -> (w1451:dbl)
            n914 = case shown="True" w1449 {
              tunnel: w1451 -> [w1457 w1471]
              tunnel: w1450 -> [w1454 w1470]
              frame False {
                n915 = flat-sequence {
                  tunnel: w1454 -> [w1458]
                  tunnel: [w1458] -> w1455
                  tunnel: w1457 -> [_]
                  tunnel: [w1461] -> w1456
                  tunnel: w1455 -> [w1461]
                  tunnel: w1456 -> [w1462]
                  tunnel: [w1462] -> w1452
                  tunnel: [w1464] -> w1453
                  tunnel: w1452 -> [w1464]
                  tunnel: w1453 -> [w1466]
                  frame #0 {
                    n916 = call "Write to pump.vi"("string"="enter pump1", "VISA resource name"=w1458) -> ()  [unwired: 1 out]
                  }
                  frame #1 {
                    n917 = Wait (ms)(milliseconds to wait="Pump pause delay (ms)") -> ()  [unwired: 1 out]
                  }
                  frame #2 {
                    n918 = call "Write to pump.vi"("string"="stop", "VISA resource name"=w1462) -> ()  [unwired: 1 out]
                  }
                  frame #3 {
                    n919 = Wait (ms)(milliseconds to wait=u32 500) -> ()  [unwired: 1 out]
                  }
                  frame #4 {
                    n920 = call "Write to pump.vi"("string"="stop", "VISA resource name"=w1466) -> ()  [unwired: 1 out]
                  }
                }
              }
              frame True {
                n921 = flat-sequence {
                  tunnel: w1470 -> [w1480]
                  tunnel: w1471 -> [w1475]
                  tunnel: w1471 -> [w1482]
                  tunnel: w1470 -> [w1483]
                  tunnel: [w1483] -> w1468
                  tunnel: [w1485] -> w1469
                  tunnel: w1468 -> [w1485]
                  tunnel: w1469 -> [w1487]
                  frame #0 {
                    n922 = local read "All Pump Parameters"() -> (w1474:T6)
                    n923 = Unbundle By Name(w1474) -> ("Pump 1"=w1481:T33)
                    n924 = call "Set pump parameters.vi"("Pump write delay (ms)"=w1475, "Volume (uL)"="Ch 2 Inject Volume (uL)", "Rate (uL/h)"="Ch 1 Inject Rate (ul/h)", "Units"=4.0, "Pump #"=1.0, "Pump Parameters In"=w1481, "VISA resource name"=w1480) -> ("Pump Parameters Out"=w1473:T33)  [unwired: 3 in]
                    n925 = Bundle By Name(cluster=w1474, "Pump 1"=w1473) -> (w1472:T6)
                    n926 = local write "All Pump Parameters"(w1472) -> ()
                  }
                  frame #1 {
                    n927 = Wait (ms)(milliseconds to wait=w1482) -> ()  [unwired: 1 out]
                  }
                  frame #2 {
                    n928 = call "Write to pump.vi"("string"="start", "VISA resource name"=w1483) -> ()  [unwired: 1 out]
                  }
                  frame #3 {
                    n929 = Wait (ms)(milliseconds to wait=u32 500) -> ()  [unwired: 1 out]
                  }
                  frame #4 {
                    n930 = call "Write to pump.vi"("string"="start", "VISA resource name"=w1487) -> ()  [unwired: 1 out]
                  }
                }
              }
            }
          }
          frame Enabled {
            n931 = call "hamilton_controller.vi"("Open?"=w1489, "valve"=enum16{"A", "B", "C", "D", "ALL"}."B", "action"=T21."MOVE VALVE") -> ()  [unwired: 8 in, 1 out]
          }
        }
      }
      event "Main:": Value Change {
        n932 = event-data() -> ()  [unwired: 7 out]
        n933 = disable-structure shown="Disabled" {
          disable-tunnel: "Main:" -> [_ w1533]
          frame Disabled {
            n934 = local read "Pump write delay (ms)"() -> (w1494:dbl)
            n935 = case shown="False" w1495 {
              tunnel: w1494 -> [w1501 w1515]
              tunnel: "Chemyx Syringe Pump Serial Port" -> [w1498 w1514]
              frame False {
                n936 = flat-sequence {
                  tunnel: w1498 -> [w1502]
                  tunnel: [w1502] -> w1499
                  tunnel: w1501 -> [_]
                  tunnel: [w1505] -> w1500
                  tunnel: w1499 -> [w1505]
                  tunnel: w1500 -> [w1506]
                  tunnel: [w1506] -> w1496
                  tunnel: [w1508] -> w1497
                  tunnel: w1496 -> [w1508]
                  tunnel: w1497 -> [w1510]
                  frame #0 {
                    n937 = call "Write to pump.vi"("string"="enter pump3", "VISA resource name"=w1502) -> ()  [unwired: 1 out]
                  }
                  frame #1 {
                    n938 = local read "Pump pause delay (ms)"() -> (w1504:u32)
                    n939 = Wait (ms)(milliseconds to wait=w1504) -> ()  [unwired: 1 out]
                  }
                  frame #2 {
                    n940 = call "Write to pump.vi"("string"="stop", "VISA resource name"=w1506) -> ()  [unwired: 1 out]
                  }
                  frame #3 {
                    n941 = Wait (ms)(milliseconds to wait=u32 0) -> ()  [unwired: 1 out]
                  }
                  frame #4 {
                    n942 = call "Write to pump.vi"("string"="stop", "VISA resource name"=w1510) -> ()  [unwired: 1 out]
                  }
                }
              }
              frame True {
                n943 = flat-sequence {
                  tunnel: w1514 -> [w1524]
                  tunnel: w1515 -> [w1519]
                  tunnel: w1515 -> [w1526]
                  tunnel: w1514 -> [w1527]
                  tunnel: [w1527] -> w1512
                  tunnel: [w1530] -> w1513
                  tunnel: w1512 -> [w1530]
                  tunnel: w1513 -> [w1531]
                  frame #0 {
                    n944 = local read "All Pump Parameters"() -> (w1518:T6)
                    n945 = Unbundle By Name(w1518) -> ("Pump 3"=w1525:T33)
                    n946 = call "Set pump parameters.vi"("Pump write delay (ms)"=w1519, "Volume (uL)"="Ch 3 Inject Volume (uL)", "Rate (uL/h)"="Ch 3 Inject Rate (ul/h)", "Units"=4.0, "Pump #"=3.0, "Pump Parameters In"=w1525, "VISA resource name"=w1524) -> ("Pump Parameters Out"=w1517:T33)  [unwired: 3 in]
                    n947 = Bundle By Name(cluster=w1518, "Pump 3"=w1517) -> (w1516:T6)
                    n948 = local write "All Pump Parameters"(w1516) -> ()
                  }
                  frame #1 {
                    n949 = Wait (ms)(milliseconds to wait=w1526) -> ()  [unwired: 1 out]
                  }
                  frame #2 {
                    n950 = call "Write to pump.vi"("string"="start", "VISA resource name"=w1527) -> ()  [unwired: 1 out]
                  }
                  frame #3 {
                    n951 = Wait (ms)(milliseconds to wait=u32 500) -> ()  [unwired: 1 out]
                  }
                  frame #4 {
                    n952 = call "Write to pump.vi"("string"="start", "VISA resource name"=w1531) -> ()  [unwired: 1 out]
                  }
